vi "Main.vi"(0 "Schritt Wegplaner":enum16{""}(ring), 1 "Schritt Status":enum16{""}(ring), 2 "Schritt Greifer":enum16{""}(ring), 3 "Schritt Umgebungserkennung":enum16{""}(ring), 4 "Schritt Geschwindigkeitsregelung":enum16{""}(ring), 5 "Schritt Pfadvefrolgung":enum16{""}(ring)) -> (14 "Haupt-VI-Enum Ausgang":T1=enum."AUS")   [LabVIEW 2019]
doc: "In dem Main-VI werden die einzelnen Schrittdaten der Teilsystem ausgewertet und sie dient als Befehls- und Taktgeber für die anderen Teilsysteme. Das Main-VI gibt nur Hauptschrittdaten heraus und wertet nur hereinkommende Schritte aus. Sensor- oder Karten-Daten werden direkt von den Teilsystem-VI verarbeitet."
uses:
  Haupt-VI-Enum.ctl
panel:
  in  "Haupt-VI-Enum Eingang":T1=enum."AUS"
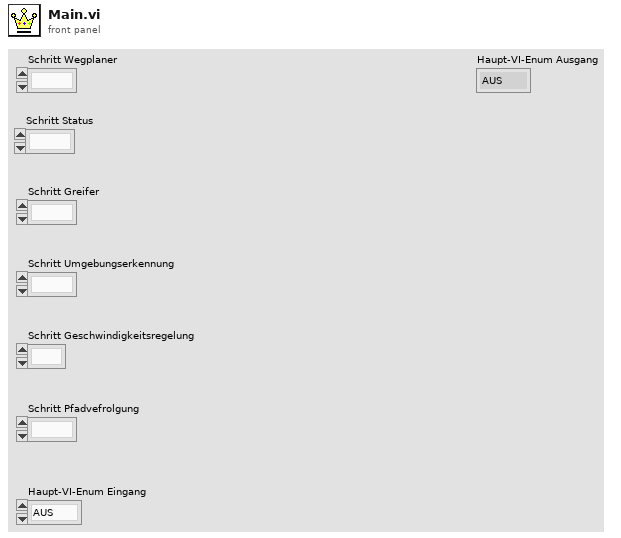
[diagram p1: front panel]
types:
  T1 = typedef "Haupt-VI-Enum.ctl" = enum16{"0 Res.", "AUS", "INIT", "Weg_planen", "Fahrfreigabe_vorwaerts", "5 Res.", "6 Res.", "7 Res.", "8 Res.", "9 Res.", "10 Res.", "Drehen", "Fahrfreigabe_Rueckwaerts", "Paketsuche", "Barcode_Paket_nicht_erkannt", "Paket_anfahren", "Paket_greifen", "17 Res.", "18 Res.", "19 Res.", "20 Res.", "Planen_vorherige_Kreuzung", "Fahrfreigabe_vorherige_Kreuzung", "Strasse_loeschen", "24 Res.", "25 Res.", "26 Res.", "27 Res.", "28 Res.", "29 Res.", "30 Res.", "Ausrichten_Poststelle", "Poststelle_Neuausrichtung", "Barcode_Poststelle_erkennt", "34 Res.", "35. Res.", "36 Res.", "37 Res.", "38 Res.", "39 Res.", "40 Res.", "Paket_abladen", "42 Res. "}
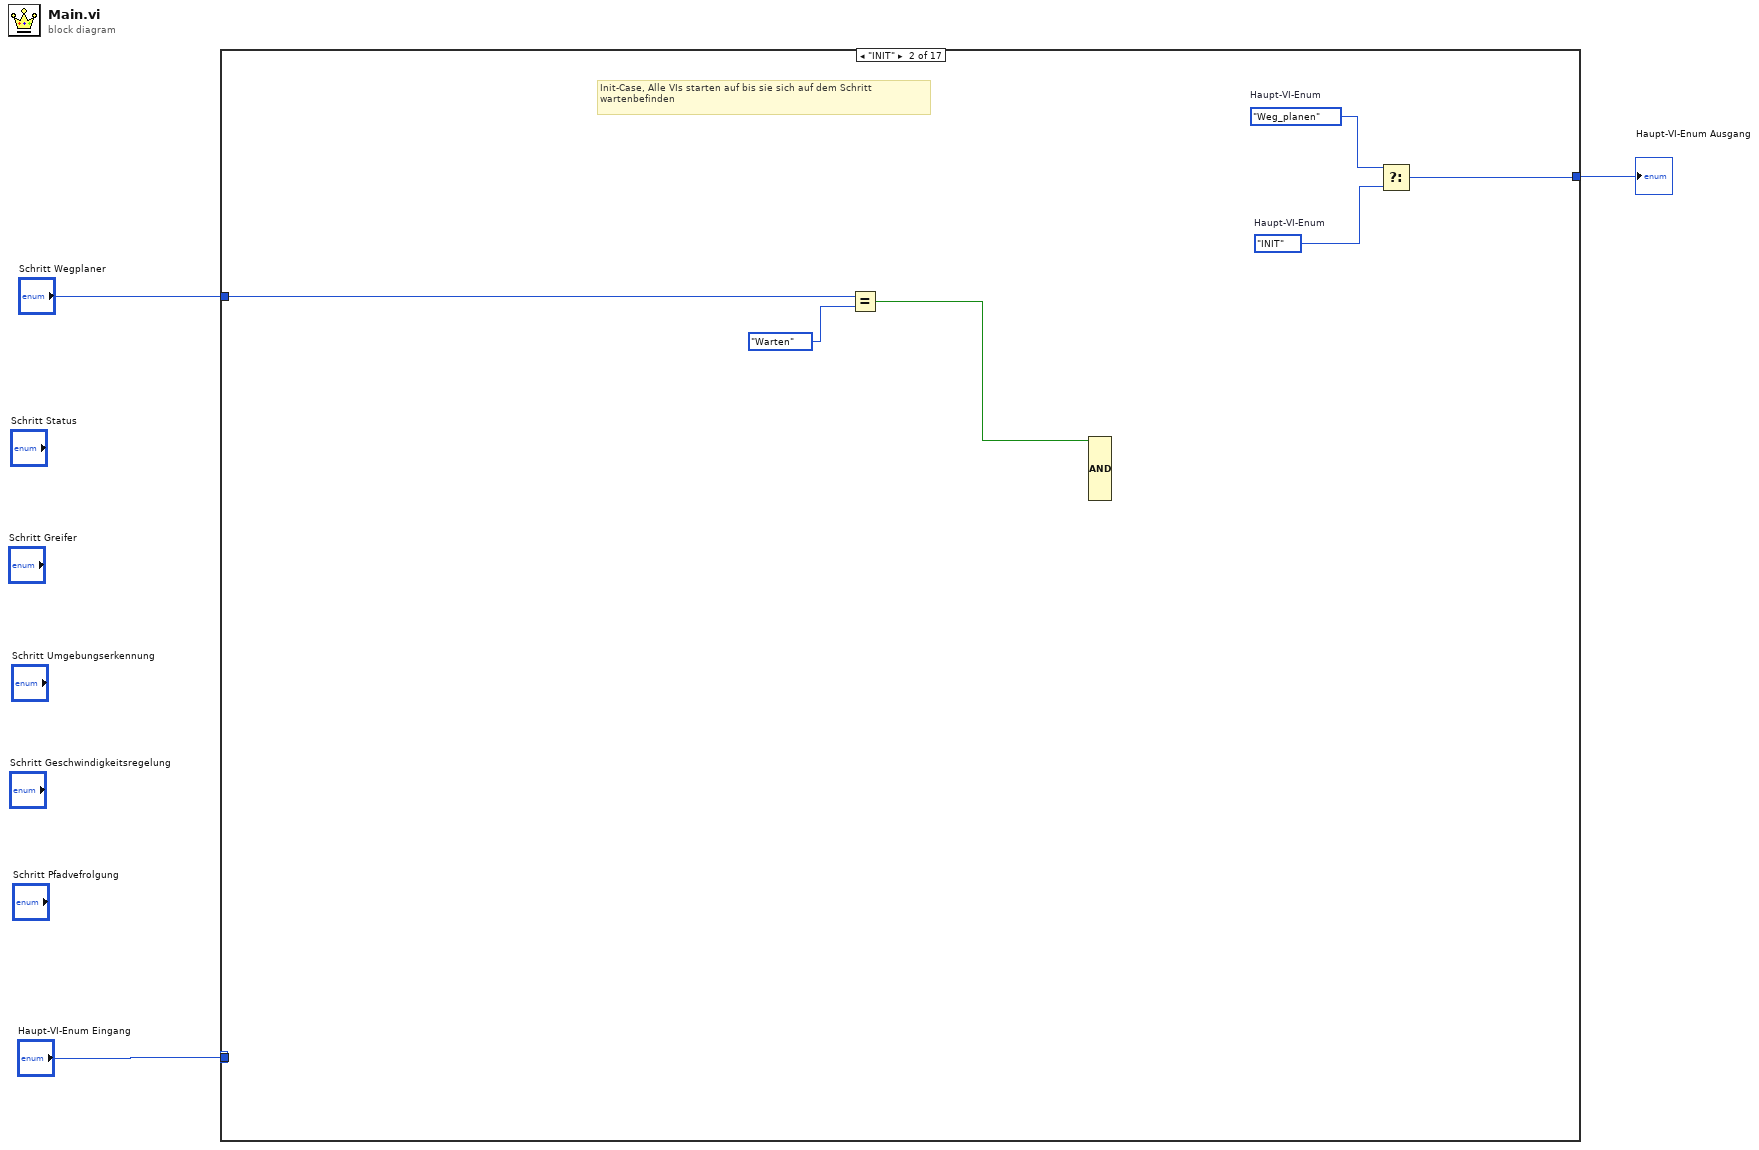
[diagram p0: block diagram]
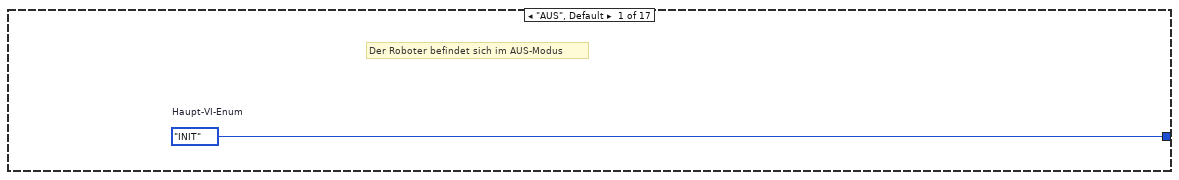
[diagram p2: hidden frame]
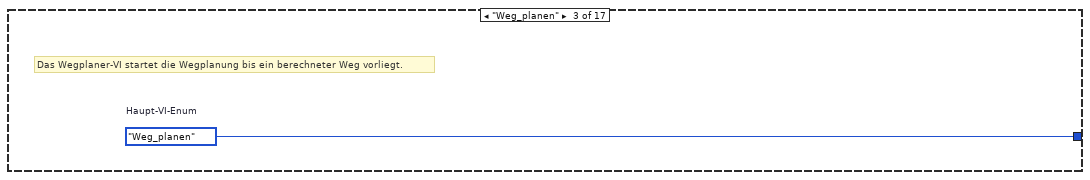
[diagram p3: hidden frame]
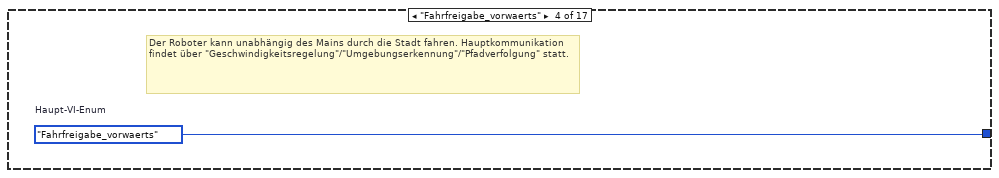
[diagram p4: hidden frame]
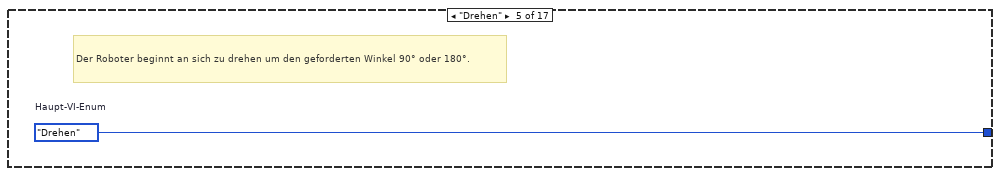
[diagram p5: hidden frame]
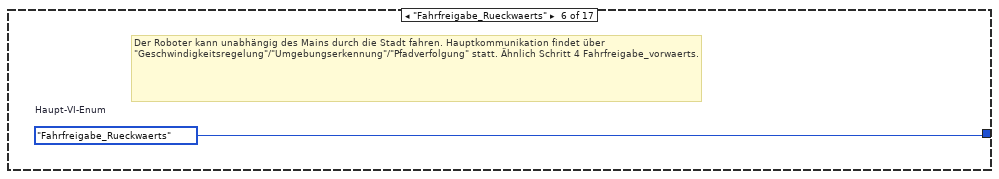
[diagram p6: hidden frame]
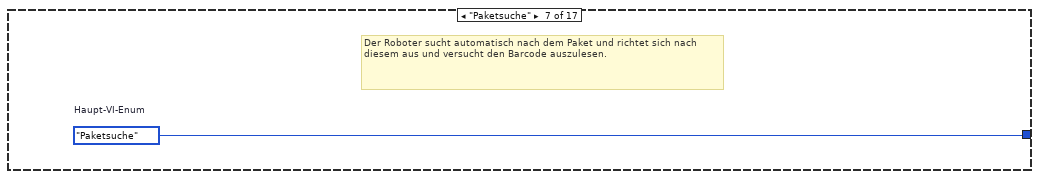
[diagram p7: hidden frame]
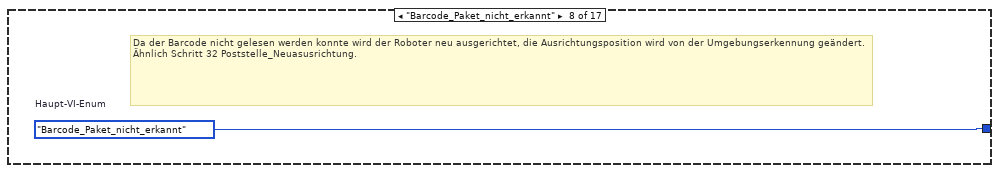
[diagram p8: hidden frame]
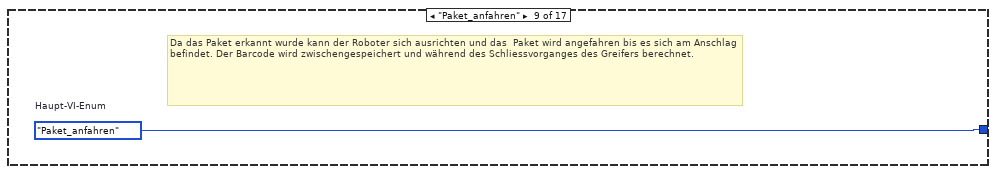
[diagram p9: hidden frame]
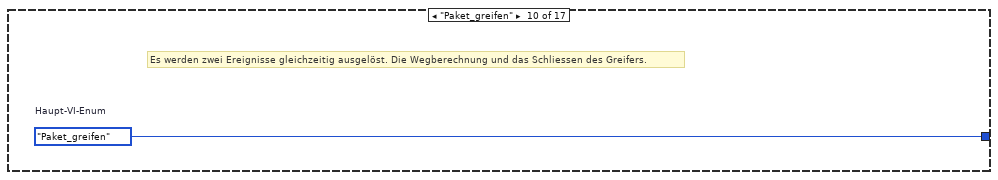
[diagram p10: hidden frame]
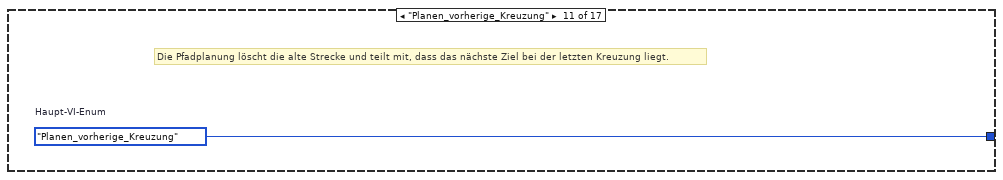
[diagram p11: hidden frame]
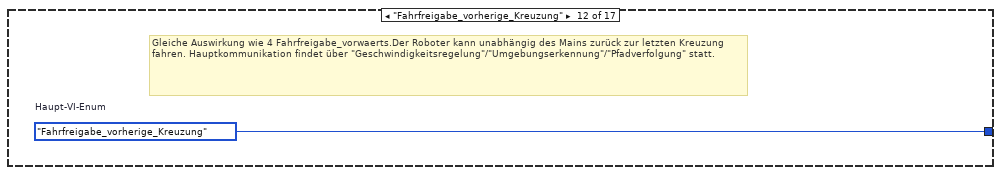
[diagram p12: hidden frame]
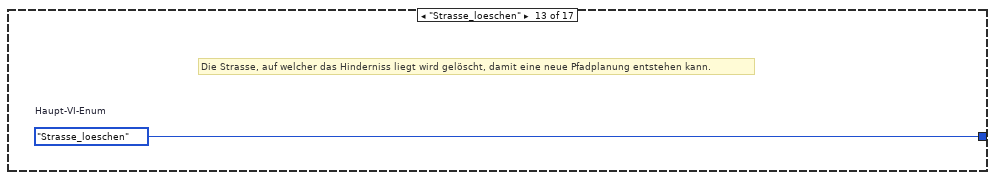
[diagram p13: hidden frame]
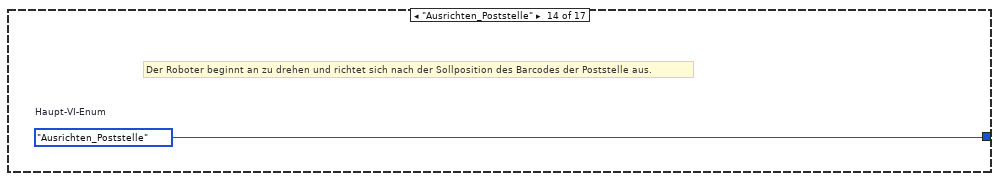
[diagram p14: hidden frame]
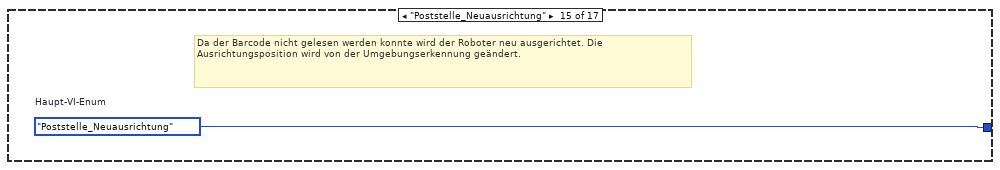
[diagram p15: hidden frame]
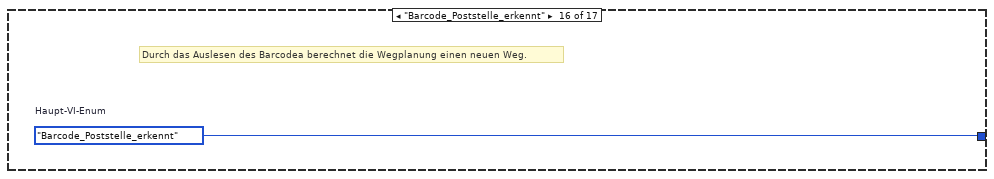
[diagram p16: hidden frame]
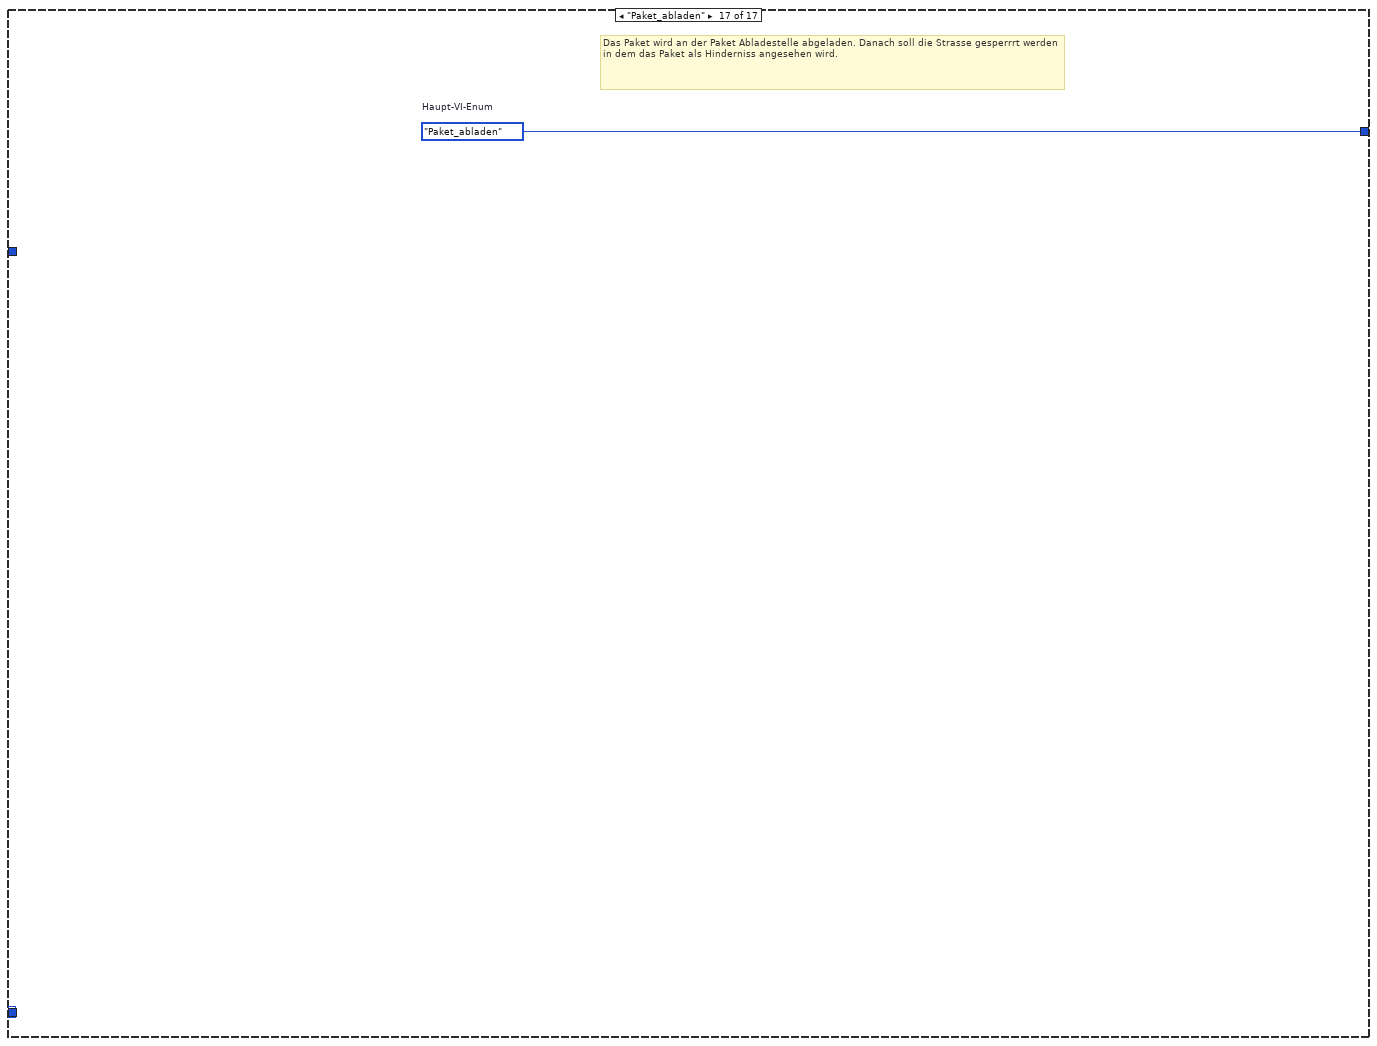
[diagram p17: hidden frame]
diagram:
  n1 = case "Case-Struktur" shown="\"INIT\"" "Haupt-VI-Enum Eingang" {
    selector: "Haupt-VI-Enum Eingang" -> [_ _ _ _ _ _ _ _ _ _ _ _ _ _ _ _ w25]
    tunnel: [w4 w10 w11 w12 w13 w14 w15 w16 w17 w18 w19 w20 w21 w22 w23 w24 w26] -> w3
    tunnel: [_ _ _ _ _ _ _ _ _ _ _ _ _ _ _ _ w25] -> _
    tunnel: "Schritt Wegplaner" -> [_ w6 _ _ _ _ _ _ _ _ _ _ _ _ _ _ _]
    frame "AUS", Default {
      w4 = Haupt-VI-Enum."INIT"  # Haupt-VI-Enum
      # "Der Roboter befindet sich im AUS-Modus"
    }
    frame "INIT" {
      w8 = Haupt-VI-Enum."Weg_planen"  # Haupt-VI-Enum
      w9 = Haupt-VI-Enum."INIT"  # Haupt-VI-Enum
      # "Init-Case, Alle VIs starten auf bis sie sich auf dem Schritt wartenbefinden"
      n2 = Equal?(x=w6, y=enum16{"Warten"}."Warten") -> (x = y?=w7:bool)
      n3 = Compound Arithmetic op=AND ("Mehrfacharithmetik")(w7) -> ()  [unwired: 7 in, 1 out]
      n4 = Select(t=w8, f=w9) -> (s? t:f=w10:T1)  [unwired: 1 in]
    }
    frame "Weg_planen" {
      w11 = Haupt-VI-Enum."Weg_planen"  # Haupt-VI-Enum
      # "Das Wegplaner-VI startet die Wegplanung bis ein berechneter Weg vorliegt."
    }
    frame "Fahrfreigabe_vorwaerts" {
      w12 = Haupt-VI-Enum."Fahrfreigabe_vorwaerts"  # Haupt-VI-Enum
      # "Der Roboter kann unabhängig des Mains durch die Stadt fahren. Hauptkommunikation findet über \"Geschwindigkeitsregelung\"/\"Umgebungserkennung\"/\"Pfadverfolgung\" statt."
    }
    frame "Drehen" {
      w13 = Haupt-VI-Enum."Drehen"  # Haupt-VI-Enum
      # "Der Roboter beginnt an sich zu drehen um den geforderten Winkel 90° oder 180°."
    }
    frame "Fahrfreigabe_Rueckwaerts" {
      w14 = Haupt-VI-Enum."Fahrfreigabe_Rueckwaerts"  # Haupt-VI-Enum
      # "Der Roboter kann unabhängig des Mains durch die Stadt fahren. Hauptkommunikation findet über \"Geschwindigkeitsregelung\"/\"Umgebungserkennung\"/\"Pfadverfolgung\" statt. Ähnlich Schritt 4 Fahrfreigabe_vorwaerts."
    }
    frame "Paketsuche" {
      w15 = Haupt-VI-Enum."Paketsuche"  # Haupt-VI-Enum
      # "Der Roboter sucht automatisch nach dem Paket und richtet sich nach diesem aus und versucht den Barcode auszulesen."
    }
    frame "Barcode_Paket_nicht_erkannt" {
      w16 = Haupt-VI-Enum."Barcode_Paket_nicht_erkannt"  # Haupt-VI-Enum
      # "Da der Barcode nicht gelesen werden konnte wird der Roboter neu ausgerichtet, die Ausrichtungsposition wird von der Umgebungserkennung geändert. Ähnlich Schritt 32 Poststelle_Neuasusrichtung."
    }
    frame "Paket_anfahren" {
      w17 = Haupt-VI-Enum."Paket_anfahren"  # Haupt-VI-Enum
      # "Da das Paket erkannt wurde kann der Roboter sich ausrichten und das  Paket wird angefahren bis es sich am Anschlag befindet. Der Barcode wird zwischengespeichert und während des Schliessvorganges des Greifers berechnet."
    }
    frame "Paket_greifen" {
      w18 = Haupt-VI-Enum."Paket_greifen"  # Haupt-VI-Enum
      # "Es werden zwei Ereignisse gleichzeitig ausgelöst. Die Wegberechnung und das Schliessen des Greifers."
    }
    frame "Planen_vorherige_Kreuzung" {
      w19 = Haupt-VI-Enum."Planen_vorherige_Kreuzung"  # Haupt-VI-Enum
      # "Die Pfadplanung löscht die alte Strecke und teilt mit, dass das nächste Ziel bei der letzten Kreuzung liegt."
    }
    frame "Fahrfreigabe_vorherige_Kreuzung" {
      w20 = Haupt-VI-Enum."Fahrfreigabe_vorherige_Kreuzung"  # Haupt-VI-Enum
      # "Gleiche Auswirkung wie 4 Fahrfreigabe_vorwaerts.Der Roboter kann unabhängig des Mains zurück zur letzten Kreuzung fahren. Hauptkommunikation findet über \"Geschwindigkeitsregelung\"/\"Umgebungserkennung\"/\"Pfadverfolgung\" statt."
    }
    frame "Strasse_loeschen" {
      w21 = Haupt-VI-Enum."Strasse_loeschen"  # Haupt-VI-Enum
      # "Die Strasse, auf welcher das Hinderniss liegt wird gelöscht, damit eine neue Pfadplanung entstehen kann."
    }
    frame "Ausrichten_Poststelle" {
      w22 = Haupt-VI-Enum."Ausrichten_Poststelle"  # Haupt-VI-Enum
      # "Der Roboter beginnt an zu drehen und richtet sich nach der Sollposition des Barcodes der Poststelle aus."
    }
    frame "Poststelle_Neuausrichtung" {
      w23 = Haupt-VI-Enum."Poststelle_Neuausrichtung"  # Haupt-VI-Enum
      # "Da der Barcode nicht gelesen werden konnte wird der Roboter neu ausgerichtet. Die Ausrichtungsposition wird von der Umgebungserkennung geändert."
    }
    frame "Barcode_Poststelle_erkennt" {
      w24 = Haupt-VI-Enum."Barcode_Poststelle_erkennt"  # Haupt-VI-Enum
      # "Durch das Auslesen des Barcodea berechnet die Wegplanung einen neuen Weg."
    }
    frame "Paket_abladen" {
      w26 = Haupt-VI-Enum."Paket_abladen"  # Haupt-VI-Enum
      # "Das Paket wird an der Paket Abladestelle abgeladen. Danach soll die Strasse gesperrrt werden in dem das Paket als Hinderniss angesehen wird."
    }
  }
  "Haupt-VI-Enum Ausgang" <- w3
